vi "Output Snip.vi"() -> ()   [LabVIEW 2015]
uses:
  request/request.lvclass/request.ctl
  <vilib>/addons/lv-msgpack/MsgPack Deserializer/Unflatten From MessagePack.vi
  output/Output.lvclass
  request/request.lvclass
panel:
  in  "Stop Button":bool
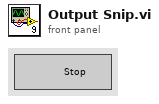
[diagram p1: front panel]
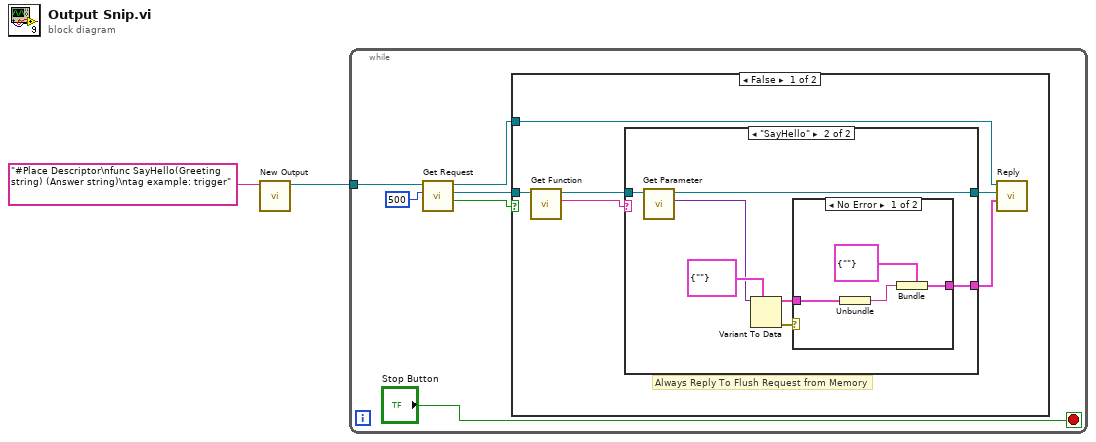
[diagram p0: block diagram]
diagram:
  n1 = call "New Output.vi"("Descriptor"="#Place Descriptor\nfunc SayHello(Greeting string) (Answer string)\ntag example: trigger") -> ("output"=w1:refnum<class "Output.lvclass">)  [unwired: 9 in, 1 out]
  n2 = while {
    tunnel: w1 -> [w7]
    stop <- "Stop Button" stop-if-true
    n3 = call "Get Request.vi"("timeout in ms (-1)"=500, "output in"=w7) -> ("timed out?"=w5:bool, "request.lvclass"=w4:refnum<class "request.lvclass">, "output out"=w3:refnum<class "Output.lvclass">)  [unwired: 6 in, 1 out]
    n4 = case shown="False" w5 {
      tunnel: w4 -> [w14 _]
      tunnel: w3 -> [w12 _]
      frame False {
        # "Always Reply To Flush Request from Memory"
        n5 = call "Get Function.vi"("request in"=w14) -> ("function"=w13:string, "request out"=w11:refnum<class "request.lvclass">)  [unwired: 8 in, 1 out]
        n6 = case shown="\"SayHello\"" w13 {
          tunnel: w11 -> [w15 w22]
          tunnel: [w15 w17] -> w10
          tunnel: [_ w18] -> w9
          frame "False", Default {
          }
          frame "SayHello" {
            n7 = call "Get Parameter.vi"("request in"=w22) -> ("parameter"=w20:variant, "request out"=w17:refnum<class "request.lvclass">)  [unwired: 8 in, 1 out]
            n8 = Variant To Data(type=cluster{"Greeting":string} {"Greeting"=""}, Variant=w20) -> (data=w19:cluster{"Greeting":string}, error out=w16:errorcluster)  [unwired: 1 in]
            n9 = case shown="No Error" w16 {
              tunnel: w19 -> [w26 _]
              tunnel: [w23 _] -> w18
              frame No Error {
                n10 = Unbundle(w26) -> ("Greeting"=w25:string)
                n11 = Bundle(cluster=cluster{"Answer":string} {"Answer"=""}, "Answer"=w25) -> (w23:cluster{"Answer":string})
              }
              frame Error {
              }
            }
          }
        }
        n12 = call "Reply.vi"("parameter"=w9, "request"=w10, "output in"=w12) -> ()  [unwired: 7 in, 2 out]
      }
      frame True {
      }
    }
  }
